vi "report results.vi"(8 "error in":errorcluster, 10 "result":refnum<class "result.lvclass">, 11 "null reporter in":refnum<class "null reporter.lvclass">) -> (0 "error out":errorcluster, 3 "null reporter out":refnum<class "null reporter.lvclass">)   [LabVIEW 2013, in "null reporter.lvclass"]
uses:
  null reporter.lvclass
  result/result.lvclass
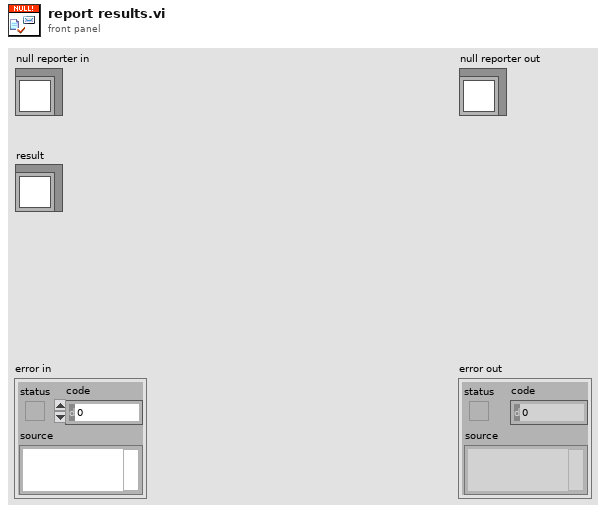
[diagram p1: front panel]
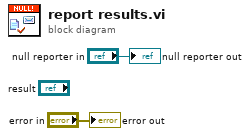
[diagram p0: block diagram]
diagram:
  "error out" <- "error in"
  "null reporter out" <- "null reporter in"
